vi "UHR-Fleezers Control (host) - 10.9.vi"() -> ()   [LabVIEW 2011] (continued)
                  n362 = local read "Oscillate Set 1"() -> (w595:bool)
                  n363 = local read "Stop All"() -> (w593:bool)
                  n364 = Or(x=w595, y=w590) -> (x .or. y?=w592:bool)
                  n365 = Not(x=w592) -> (.not. x?=w594:bool)
                  n366 = Compound Arithmetic op=OR(w593, w594) -> (w591:bool)
                }
              }
              n367 = node-c288() -> ()  [unwired: 2 out]
            }
            n368 = node-c288(w436) -> ()  [unwired: 1 out]
          }
        }
      }
      event "Fl. Triggered...": Value Change {
        n369 = event-data() -> ()  [unwired: 7 out]
        n370 = case shown="True" "Fl. Triggered..." {
          frame False {
          }
          frame True {
            n371 = node-c288() -> (w606:T21)  [unwired: 4 out]
            n372 = timed-loop {
              timing: w606 -> [_]
              timing-out: [_] -> w605
              tunnel: "Action" -> [w614]
              shift-right: [w611] -> _
              shift-left: u8 255 -> [w613]
              shift-right: [w608] -> _
              shift-left: 255 -> [w610]
              stop <- w607 stop-if-true
              n373 = node-c288() -> ()  [unwired: 2 out]
              n374 = flat-sequence {
                tunnel: w614 -> [w631]
                tunnel: w613 -> [w630]
                tunnel: [w629] -> w612
                tunnel: w610 -> [w616]
                tunnel: [w615] -> w609
                tunnel: [w911] -> w607
                tunnel: w612 -> [w910]
                tunnel: [w910] -> w611
                tunnel: [w909] -> w608
                tunnel: w609 -> [w909]
                frame #0 {
                  n375 = local read "Delta Fl. 2"() -> (w628:dbl)
                  n376 = local read "Delta Fl. 1"() -> (w623:dbl)
                  n377 = Multiply(x="Fl. Delta Thresh. (kHz)", y=1000.0) -> (x*y=w618:dbl)
                  n378 = Select(t=w623, s="APD to Watch", f=w628) -> (s? t:f=w619:dbl)
                  n379 = Greater?(x=w619, y=w618) -> (0:w624:bool)
                  n380 = Or(x="Force Yank", y=w624) -> (x .or. y?=w622:bool)
                  n381 = And(x=w622, y="Yank when bind or unbind?") -> (x .and. y?=w620:bool)
                  n382 = case shown="False" w620 {
                    tunnel: w631 -> [w633 w785]
                    tunnel: w630 -> [w635 w781]
                    tunnel: [w635 w778] -> w629
                    tunnel: w619 -> [w641 _]
                    tunnel: w618 -> [w640 _]
                    tunnel: "Force Yank" -> [w638 _]
                    tunnel: w616 -> [w637 w777]
                    tunnel: [w636 w777] -> w615
                    frame False {
                      n383 = Negate(x=w640) -> (-x=w632:dbl)
                      n384 = Less?(x=w641, y=w632) -> (x < y?=w639:bool)
                      n385 = Or(x=w638, y=w639) -> (x .or. y?=w634:bool)
                      n386 = case shown="True" w634 {
                        tunnel: w637 -> [w642 w652]
                        tunnel: [w642 w651] -> w636
                        tunnel: w633 -> [_ w650]
                        frame False {
                        }
                        frame True {
                          n387 = flat-sequence {
                            tunnel: w652 -> [w658]
                            tunnel: w650 -> [w655]
                            tunnel: [w657] -> w649
                            tunnel: [w656] -> w648
                            tunnel: [w655] -> w647
                            tunnel: w646 -> [w654]
                            tunnel: [w654] -> w645
                            tunnel: w644 -> [w653]
                            tunnel: [w653] -> w643
                            tunnel: [w704] -> w651
                            tunnel: w649 -> [w704]
                            tunnel: w648 -> [w703]
                            tunnel: w647 -> [w702]
                            tunnel: w645 -> [w701]
                            tunnel: w643 -> [w700]
                            frame #0 {
                              n388 = call <vilib>:"Beep.vi"() -> ()  [unwired: 12 in]
                              n389 = local write "Waiting"(FALSE ("Waiting")) -> ()
                              n390 = Increment(x=w658) -> (x+1=w657:i32)
                              n391 = case shown="\"Yank\"" w655 {
                                tunnel: w657 -> [_ w663 _]
                                frame "Alarm", Default {
                                }
                                frame "Yank" {
                                n392 = flat-sequence {
                                tunnel: w663 -> [w666]
                                tunnel: [w665] -> w662
                                tunnel: [w664] -> w661
                                tunnel: w662 -> [w676]
                                tunnel: w661 -> [w677]
                                frame #0 {
                                n393 = local read "Yank Delay (s)"() -> (w669:dbl)
                                n394 = local read "N Array El"() -> (w664:u8)
                                n395 = Quotient & Remainder(x=w666, y=w664) -> (x-y*floor(x/y)=w665:i32)  [unwired: 1 out]
                                n396 = Multiply(x=w669, y=1000.0) -> (x*y=w667:dbl)
                                n397 = Wait (ms)(milliseconds to wait=w667) -> ()  [unwired: 1 out]
                                }
                                frame #1 {
                                n398 = local read "Yank to which?"() -> (w671:bool)
                                n399 = local read "Random Choice"() -> (w681:bool)
                                n400 = local read "Yank to Delta Array (MHz)"() -> (w674:dbl[])
                                n401 = local read "Yank to SP"() -> (w675:dbl[])
                                n402 = Random Number (0-1)() -> (number: 0 to 1=w680:dbl)
                                n403 = Multiply(x=w677, y=w680) -> (x*y=w679:dbl)
                                n404 = Round Toward -Infinity(1:w679) -> (0:w678:dbl)
                                n405 = Select(t=w678, s=w681, f=w676) -> (s? t:f=w672:dbl)
                                n406 = Select(t=w674, s=w671, f=w675) -> (s? t:f=w673:dbl[])
                                n407 = Index Array(array=w673, index=w672) -> (element=w670:dbl)
                                n408 = case shown="False" w671 {
                                tunnel: w670 -> [w682 w697]
                                frame False {
                                n409 = flat-sequence {
                                tunnel: w682 -> [w683]
                                frame #0 {
                                n410 = property on="Trap Pos FB SP" class="DigNum (strict)"("Val(Sgnl)"=w683) -> ()  [unwired: 2 in, 2 out]
                                }
                                frame #1 {
                                n411 = Wait (ms)(milliseconds to wait=u32 700) -> ()  [unwired: 1 out]
                                }
                                frame #2 {
                                n412 = local read "Action (%)"() -> (w688:dbl)
                                n413 = Absolute Value(x=w688) -> (abs(x)=w687:dbl)
                                n414 = Greater?(x=w687, y=70.0) -> (0:w685:bool)
                                n415 = property on="Remove Action Offset" class="Bool (strict)"("Val(Sgnl)"=w685) -> ()  [unwired: 2 in, 2 out]
                                }
                                frame #3 {
                                n416 = for {
                                N: 4 -> [_]
                                n417 = flat-sequence {
                                frame #0 {
                                n418 = Wait (ms)(milliseconds to wait=u32 500) -> ()  [unwired: 1 out]
                                }
                                frame #1 {
                                n419 = local read "Action (%)"() -> (w694:dbl)
                                n420 = Absolute Value(x=w694) -> (abs(x)=w693:dbl)
                                n421 = Greater?(x=w693, y=70.0) -> (0:w691:bool)
                                n422 = property on="Remove Action Offset" class="Bool (strict)"("Val(Sgnl)"=w691) -> ()  [unwired: 2 in, 2 out]
                                }
                                }
                                }
                                }
                                frame #4 {
                                n423 = Wait (ms)(milliseconds to wait=u32 1500) -> ()  [unwired: 1 out]
                                }
                                frame #5 {
                                n424 = property on="Rem fb disp offset" class="Bool (strict)"("Val(Sgnl)"=TRUE ("Value (Signaling)")) -> ()  [unwired: 2 in, 2 out]
                                }
                                }
                                }
                                frame True {
                                n425 = property on="Trap Delta (MHz)" class="DigNum (strict)"("Val(Sgnl)"=w697) -> ()  [unwired: 2 in, 2 out]
                                }
                                }
                                }
                                }
                                }
                                frame "Image" {
                                n426 = property on="Confocal Image" class="Bool (strict)"("Val(Sgnl)"=TRUE ("Value (Signaling)")) -> ()  [unwired: 2 in, 2 out]
                                }
                              }
                              n427 = local write "Fl. High"(FALSE ("Fl. High")) -> ()
                              n428 = local read "Time (s)"() -> (w656:dbl)
                            }
                            frame #1 {
                              n429 = case shown="True" "Auto F Reset" {
                                tunnel: w703 -> [_ w708]
                                tunnel: w702 -> [_ w707]
                                tunnel: w701 -> [_ w706]
                                tunnel: w700 -> [_ w705]
                                frame False {
                                }
                                frame True {
                                n430 = node-c288() -> (w710:T21)  [unwired: 4 in]
                                n431 = timed-loop {
                                timing: w710 -> [_]
                                timing-out: [_] -> w709
                                tunnel: w708 -> [w715]
                                tunnel: w707 -> [w714]
                                tunnel: w706 -> [w713]
                                tunnel: w705 -> [w712]
                                stop <- w711 stop-if-true
                                n432 = node-c288() -> ()  [unwired: 1 in, 1 out]
                                n433 = local read "Fl. Delta Thresh. (kHz)"() -> (w724:dbl)
                                n434 = local read "APD to Watch"() -> (w725:bool)
                                n435 = local read "Delta Fl. 1"() -> (w726:dbl)
                                n436 = local read "Delta Fl. 2"() -> (w727:dbl)
                                n437 = local read "Fl. Triggered..."() -> (w718:bool)
                                n438 = local read "Stop All"() -> (w719:bool)
                                n439 = local read "Force Reset"() -> (w717:bool)
                                n440 = Multiply(x=w724, y=1000.0) -> (x*y=w722:dbl)
                                n441 = Not(x=w718) -> (.not. x?=w716:bool)
                                n442 = Select(t=w726, s=w725, f=w727) -> (s? t:f=w721:dbl)
                                n443 = Greater?(x=w721, y=w722) -> (0:w720:bool)
                                n444 = Compound Arithmetic op=OR(w720, w719, w716, w717) -> (w711:bool)
                                n445 = case shown="True" w711 {
                                tunnel: w715 -> [_ w731]
                                tunnel: w714 -> [_ w735]
                                tunnel: w713 -> [_ w734]
                                tunnel: w712 -> [_ w733]
                                frame False {
                                }
                                frame True {
                                n446 = case shown="\"Yank\"" w735 {
                                tunnel: w734 -> [_ w745]
                                tunnel: w733 -> [_ w743]
                                frame "Image", Default {
                                }
                                frame "Yank" {
                                n447 = flat-sequence {
                                tunnel: [w748] -> w746
                                tunnel: w745 -> [w748]
                                tunnel: [w747] -> w744
                                tunnel: w743 -> [w747]
                                tunnel: w746 -> [w754]
                                tunnel: w744 -> [w752]
                                frame #0 {
                                n448 = local read "Yank Delay (s)"() -> (w751:dbl)
                                n449 = Multiply(x=w751, y=1000.0) -> (x*y=w749:dbl)
                                n450 = Wait (ms)(milliseconds to wait=w749) -> ()  [unwired: 1 out]
                                }
                                frame #1 {
                                n451 = local read "Yank to which?"() -> (w753:bool)
                                n452 = case shown="False" w753 {
                                tunnel: w754 -> [_ w770]
                                tunnel: w752 -> [w755 _]
                                frame False {
                                n453 = flat-sequence {
                                tunnel: w755 -> [w756]
                                frame #0 {
                                n454 = property on="Trap Pos FB SP" class="DigNum (strict)"("Val(Sgnl)"=w756) -> ()  [unwired: 2 in, 2 out]
                                }
                                frame #1 {
                                n455 = Wait (ms)(milliseconds to wait=u32 700) -> ()  [unwired: 1 out]
                                }
                                frame #2 {
                                n456 = local read "Action (%)"() -> (w761:dbl)
                                n457 = Absolute Value(x=w761) -> (abs(x)=w760:dbl)
                                n458 = Greater?(x=w760, y=70.0) -> (0:w758:bool)
                                n459 = property on="Remove Action Offset" class="Bool (strict)"("Val(Sgnl)"=w758) -> ()  [unwired: 2 in, 2 out]
                                }
                                frame #3 {
                                n460 = for {
                                N: 4 -> [_]
                                n461 = flat-sequence {
                                frame #0 {
                                n462 = Wait (ms)(milliseconds to wait=u32 500) -> ()  [unwired: 1 out]
                                }
                                frame #1 {
                                n463 = local read "Action (%)"() -> (w767:dbl)
                                n464 = Absolute Value(x=w767) -> (abs(x)=w766:dbl)
                                n465 = Greater?(x=w766, y=70.0) -> (0:w764:bool)
                                n466 = property on="Remove Action Offset" class="Bool (strict)"("Val(Sgnl)"=w764) -> ()  [unwired: 2 in, 2 out]
                                }
                                }
                                }
                                }
                                frame #4 {
                                n467 = Wait (ms)(milliseconds to wait=u32 1500) -> ()  [unwired: 1 out]
                                }
                                frame #5 {
                                n468 = property on="Rem fb disp offset" class="Bool (strict)"("Val(Sgnl)"=TRUE ("Value (Signaling)")) -> ()  [unwired: 2 in, 2 out]
                                }
                                }
                                }
                                frame True {
                                n469 = property on="Trap Delta (MHz)" class="DigNum (strict)"("Val(Sgnl)"=w770) -> ()  [unwired: 2 in, 2 out]
                                }
                                }
                                }
                                }
                                }
                                }
                                n470 = local read "Time (s)"() -> (w730:dbl)
                                n471 = Subtract(x=w731, y=w730) -> (x-y=w742:dbl)
                                n472 = Number To Decimal String(number=w742, width (-)=i16 0) -> (decimal integer string=w740:string)
                                n473 = Concatenate Strings(w740, " s fluorescence event") -> (w737:string)
                                n474 = local read "Messages"() -> (w738:string)
                                n475 = local write "Duration (s)"(w742) -> ()
                                n476 = call "Update messages.vi"("Message to add"=w737, "Old message string"=w738) -> ("New message string"=w736:string)
                                n477 = local write "Messages"(w736) -> ()
                                n478 = call <vilib>:"Beep.vi"() -> ()  [unwired: 12 in]
                                n479 = local write "Force Reset"(FALSE ("Force Reset")) -> ()
                                n480 = local write "Fl. High"(TRUE ("Fl. High")) -> ()
                                n481 = local write "Waiting"(TRUE ("Waiting")) -> ()
                                }
                                }
                                n482 = node-c288() -> ()  [unwired: 1 in, 1 out]
                                }
                                n483 = node-c288(w709) -> ()  [unwired: 1 out]
                                }
                              }
                            }
                          }
                          n484 = local read "Trap Delta (MHz)"() -> (w646:dbl)
                          n485 = local read "Trap Pos FB SP"() -> (w644:fxp<+/-,16,1>)
                        }
                      }
                    }
                    frame True {
                      n486 = flat-sequence {
                        tunnel: w782 -> [w792]
                        tunnel: [w792] -> w786
                        tunnel: w785 -> [w791]
                        tunnel: [w791] -> w784
                        tunnel: [w790] -> w783
                        tunnel: w781 -> [w789]
                        tunnel: [w788] -> w780
                        tunnel: w776 -> [w787]
                        tunnel: [w787] -> w775
                        tunnel: w786 -> [w838]
                        tunnel: w784 -> [w837]
                        tunnel: w783 -> [w836]
                        tunnel: w780 -> [w835]
                        tunnel: [w835] -> w779
                        tunnel: w775 -> [w834]
                        tunnel: w779 -> [w907]
                        tunnel: [w907] -> w778
                        frame #0 {
                          n487 = call <vilib>:"Beep.vi"() -> ()  [unwired: 3 in, 9 out]
                          n488 = local write "Waiting"(FALSE ("Waiting")) -> ()
                          n489 = Increment(x=w789) -> (x+1=w788:u8)
                          n490 = case shown="\"Yank\"" w791 {
                            tunnel: w788 -> [_ _ w798]
                            frame "Image" {
                              n491 = property on="Confocal Image" class="Bool (strict)"("Val(Sgnl)"=TRUE ("Value (Signaling)")) -> ()  [unwired: 2 in, 2 out]
                            }
                            frame "Alarm", Default {
                            }
                            frame "Yank" {
                              n492 = flat-sequence {
                                tunnel: w798 -> [w801]
                                tunnel: [w800] -> w797
                                tunnel: ["N Array El"] -> w796
                                tunnel: w797 -> [w815]
                                tunnel: w796 -> [w811]
                                frame #0 {
                                n493 = Multiply(x="Yank Delay (s)", y=1000.0) -> (x*y=w804:dbl)
                                n494 = Quotient & Remainder(x=w801, y="N Array El") -> (x-y*floor(x/y)=w800:u8)  [unwired: 1 out]
                                n495 = Wait (ms)(milliseconds to wait=w804) -> ()  [unwired: 1 out]
                                }
                                frame #1 {
                                n496 = Random Number (0-1)() -> (number: 0 to 1=w812:dbl)
                                n497 = Multiply(x=w811, y=w812) -> (x*y=w810:dbl)
                                n498 = Round Toward -Infinity(1:w810) -> (0:w809:dbl)
                                n499 = Select(t=w809, s="Random Choice", f=w815) -> (s? t:f=w813:dbl)
                                n500 = Select(t="Yank to Delta Array (MHz)", s="Yank to which?", f="Yank to SP") -> (s? t:f=w806:dbl[])
                                n501 = Index Array(array=w806, index=w813) -> (element=w816:dbl)
                                n502 = case shown="False" "Yank to which?" {
                                tunnel: w816 -> [w817 w832]
                                frame False {
                                n503 = flat-sequence {
                                tunnel: w817 -> [w818]
                                frame #0 {
                                n504 = property on="Trap Pos FB SP" class="DigNum (strict)"("Val(Sgnl)"=w818) -> ()  [unwired: 2 in, 2 out]
                                }
                                frame #1 {
                                n505 = Wait (ms)(milliseconds to wait=u32 700) -> ()  [unwired: 1 out]
                                }
                                frame #2 {
                                n506 = local read "Action (%)"() -> (w823:dbl)
                                n507 = Absolute Value(x=w823) -> (abs(x)=w822:dbl)
                                n508 = Greater?(x=w822, y=70.0) -> (0:w820:bool)
                                n509 = property on="Remove Action Offset" class="Bool (strict)"("Val(Sgnl)"=w820) -> ()  [unwired: 2 in, 2 out]
                                }
                                frame #3 {
                                n510 = for {
                                N: 4 -> [_]
                                n511 = flat-sequence {
                                frame #0 {
                                n512 = Wait (ms)(milliseconds to wait=u32 500) -> ()  [unwired: 1 out]
                                }
                                frame #1 {
                                n513 = local read "Action (%)"() -> (w829:dbl)
                                n514 = Absolute Value(x=w829) -> (abs(x)=w828:dbl)
                                n515 = Greater?(x=w828, y=70.0) -> (0:w826:bool)
                                n516 = property on="Remove Action Offset" class="Bool (strict)"("Val(Sgnl)"=w826) -> ()  [unwired: 2 in, 2 out]
                                }
                                }
                                }
                                }
                                frame #4 {
                                n517 = Wait (ms)(milliseconds to wait=u32 1500) -> ()  [unwired: 1 out]
                                }
                                frame #5 {
                                n518 = property on="Rem fb disp offset" class="Bool (strict)"("Val(Sgnl)"=TRUE ("Value (Signaling)")) -> ()  [unwired: 2 in, 2 out]
                                }
                                }
                                }
                                frame True {
                                n519 = property on="Trap Delta (MHz)" class="DigNum (strict)"("Val(Sgnl)"=w832) -> ()  [unwired: 2 in, 2 out]
                                }
                                }
                                }
                              }
                            }
                          }
                          n520 = local read "Time (s)"() -> (w790:dbl)
                          "Fl. High" <- TRUE ("Yanking")
                        }
                        frame #1 {
                          n521 = local read "Auto F Reset"() -> (w833:bool)
                          n522 = case shown="True" w833 {
                            tunnel: w838 -> [_ w842]
                            tunnel: w837 -> [_ w841]
                            tunnel: w836 -> [_ w840]
                            tunnel: w834 -> [_ w839]
                            frame False {
                            }
                            frame True {
                              n523 = node-c288() -> (w844:T21)  [unwired: 4 out]
                              n524 = timed-loop {
                                timing: w844 -> [_]
                                timing-out: [_] -> w843
                                tunnel: w842 -> [w862]
                                tunnel: w841 -> [w861]
                                tunnel: w840 -> [w860]
                                tunnel: w839 -> [w859]
                                stop <- w845 stop-if-true
                                n525 = node-c288() -> ()  [unwired: 2 out]
                                n526 = local read "Fl. Delta Thresh. (kHz)"() -> (w853:dbl)
                                n527 = local read "Fl. Triggered..."() -> (w858:bool)
                                n528 = local read "Delta Fl. 1"() -> (w849:dbl)
                                n529 = local read "Delta Fl. 2"() -> (w847:dbl)
                                n530 = local read "Stop All"() -> (w856:bool)
                                n531 = local read "APD to Watch"() -> (w848:bool)
                                n532 = Select(t=w849, s=w848, f=w847) -> (s? t:f=w846:dbl)
                                n533 = Not(x=w858) -> (.not. x?=w857:bool)
                                n534 = Multiply(x=w853, y=1000.0) -> (x*y=w852:dbl)
                                n535 = Negate(x=w852) -> (-x=w851:dbl)
                                n536 = Less?(x=w846, y=w851) -> (x < y?=w855:bool)
                                n537 = Compound Arithmetic op=OR(w855, w856, w857, "Force Reset") -> (w845:bool)
                                n538 = case shown="True" w845 {
                                tunnel: w862 -> [_ w874]
                                tunnel: w861 -> [_ w873]
                                tunnel: w860 -> [_ w863]
                                tunnel: w859 -> [_ w865]
                                frame False {
                                }
                                frame True {
                                n539 = case shown="\"Yank\"" w873 {
                                tunnel: w874 -> [_ w877]
                                tunnel: w865 -> [_ w875]
                                frame "Image", Default {
                                }
                                frame "Yank" {
                                n540 = flat-sequence {
                                tunnel: [w883] -> w878
                                tunnel: w877 -> [w883]
                                tunnel: [w879] -> w876
                                tunnel: w875 -> [w879]
                                tunnel: w878 -> [w886]
                                tunnel: w876 -> [w884]
                                frame #0 {
                                n541 = local read "Yank Delay (s)"() -> (w882:dbl)
                                n542 = Multiply(x=w882, y=1000.0) -> (x*y=w880:dbl)
                                n543 = Wait (ms)(milliseconds to wait=w880) -> ()  [unwired: 1 out]
                                }
                                frame #1 {
                                n544 = local read "Yank to which?"() -> (w885:bool)
                                n545 = case shown="False" w885 {
                                tunnel: w886 -> [_ w902]
                                tunnel: w884 -> [w887 _]
                                frame False {
                                n546 = flat-sequence {
                                tunnel: w887 -> [w888]
                                frame #0 {
                                n547 = property on="Trap Pos FB SP" class="DigNum (strict)"("Val(Sgnl)"=w888) -> ()  [unwired: 2 in, 2 out]
                                }
                                frame #1 {
                                n548 = Wait (ms)(milliseconds to wait=u32 700) -> ()  [unwired: 1 out]
                                }
                                frame #2 {
                                n549 = local read "Action (%)"() -> (w893:dbl)
                                n550 = Absolute Value(x=w893) -> (abs(x)=w892:dbl)
                                n551 = Greater?(x=w892, y=70.0) -> (0:w890:bool)
                                n552 = property on="Remove Action Offset" class="Bool (strict)"("Val(Sgnl)"=w890) -> ()  [unwired: 2 in, 2 out]
                                }
                                frame #3 {
                                n553 = for {
                                N: 4 -> [_]
                                n554 = flat-sequence {
                                frame #0 {
                                n555 = Wait (ms)(milliseconds to wait=u32 500) -> ()  [unwired: 1 out]
                                }
                                frame #1 {
                                n556 = local read "Action (%)"() -> (w899:dbl)
                                n557 = Absolute Value(x=w899) -> (abs(x)=w898:dbl)
                                n558 = Greater?(x=w898, y=70.0) -> (0:w896:bool)
                                n559 = property on="Remove Action Offset" class="Bool (strict)"("Val(Sgnl)"=w896) -> ()  [unwired: 2 in, 2 out]
                                }
                                }
                                }
                                }
                                frame #4 {
                                n560 = Wait (ms)(milliseconds to wait=u32 1500) -> ()  [unwired: 1 out]
                                }
                                frame #5 {
                                n561 = property on="Rem fb disp offset" class="Bool (strict)"("Val(Sgnl)"=TRUE ("Value (Signaling)")) -> ()  [unwired: 2 in, 2 out]
                                }
                                }
                                }
                                frame True {
                                n562 = property on="Trap Delta (MHz)" class="DigNum (strict)"("Val(Sgnl)"=w902) -> ()  [unwired: 2 in, 2 out]
                                }
                                }
                                }
                                }
                                }
                                }
                                n563 = local read "Time (s)"() -> (w864:dbl)
                                n564 = local read "Messages"() -> (w872:string)
                                n565 = Subtract(x=w864, y=w863) -> (x-y=w870:dbl)
                                "Duration (s)" <- w870
                                n566 = Number To Decimal String(number=w870, width (-)=i16 0) -> (decimal integer string=w868:string)
                                n567 = Concatenate Strings(w868, " s fluorescence event." ("string")) -> (w866:string)
                                n568 = call "Update messages.vi"("Message to add"=w866, "Old message string"=w872) -> ("New message string"=w871:string)
                                n569 = local write "Messages"(w871) -> ()
                                n570 = call <vilib>:"Beep.vi"() -> ()  [unwired: 3 in, 9 out]
                                }
                                }
                                n571 = node-c288() -> ()  [unwired: 2 out]
                              }
                              n572 = node-c288(w843) -> ()  [unwired: 1 out]
                            }
                          }
                        }
                        frame #2 {
                          n573 = local write "Fl. High"(FALSE ("Yanking")) -> ()
                        }
                      }
                      n574 = local read "Trap Delta (MHz)"() -> (w782:dbl)
                      n575 = local read "Trap Pos FB SP"() -> (w776:fxp<+/-,16,1>)
                    }
                  }
                }
                frame #1 {
                  n576 = local read "Stop All"() -> (w914:bool)
                  n577 = local read "Fl. Triggered..."() -> (w912:bool)
                  n578 = Not(x=w912) -> (.not. x?=w913:bool)
                  n579 = Or(x=w913, y=w914) -> (x .or. y?=w911:bool)
                  n580 = Not(x=w911) -> (.not. x?=→"Waiting":bool)
                }
              }
              n581 = node-c288() -> ()  [unwired: 2 out]
            }
            n582 = node-c288(w605) -> ()  [unwired: 1 out]
          }
        }
      }
      event "Stop All": Value Change {
        n583 = event-data() -> ()  [unwired: 7 out]
        n584 = local read "Stop All"() -> (w920:bool)
      }
    }
    n585 = node-c288() -> ()  [unwired: 2 out]
  }
  n586 = node-c288() -> (w79:T21)  [unwired: 4 in]
  n587 = node-c288(2 ("Processor")) -> (w92:T21)  [unwired: 3 out]
  n588 = timed-loop "Run Scripts, including: stage motion" {
    tunnel: w84 -> [w927]
    tunnel: w83 -> [w928]
    tunnel: [w928] -> w82
    tunnel: [w927] -> w81
    timing: w79 -> [_]
    timing-out: [_] -> w78
    tunnel: w64 -> [w926]
    tunnel: w65 -> [w925]
    tunnel: w4 -> [w922]
    tunnel: w3 -> [w921]
    tunnel: w2 -> [w923]
    tunnel: w1 -> [w924]
    stop <- w929 stop-if-true
    n589 = node-c288() -> ()  [unwired: 1 in, 1 out]
    n590 = event shown="[12] \"Force FB Data\nScript\": Value Change" {
      selector: _ -> [_ _ _ _ _ _ _ _ _ _ _ _ _ _ _ _ _ _ _]
      dyn-events: _ -> [_ _ _ _ _ _ _ _ _ _ _ _ _ _ _ _ _ _ _]
      timeout: _ -> [_ _ _ _ _ _ _ _ _ _ _ _ _ _ _ _ _ _ _]
      tunnel: ["Set Position" "Move to Position" _ _ "Read Harvard" _ _ _ _ _ _ "Got ADig bead" "Force FB Data\nScript" _ "Got DNA bead" "Take Stepping Data" _ "Take Detection Laser\nImage" _] -> _
      tunnel: [_ _ _ _ _ _ _ _ _ _ _ _ _ _ _ _ _ _ w1546] -> w929
      tunnel: w927 -> [w947 w955 w968 w998 _ w1043 w1083 w1164 w1193 w1325 w1351 _ w1387 _ _ _ _ _ _]
      tunnel: w928 -> [w948 w956 w969 w999 _ w1044 w1084 w1165 w1194 w1326 w1352 _ w1388 _ _ _ _ _ _]
      tunnel: w926 -> [_ _ _ _ w1028 _ _ _ _ _ _ _ _ _ _ _ _ _ _]
      tunnel: w925 -> [_ _ _ _ w1027 _ _ _ _ _ _ _ _ _ _ _ _ _ _]
      tunnel: w924 -> [_ _ _ _ _ _ _ _ _ _ _ _ _ _ _ _ _ _ _]
      tunnel: w923 -> [_ _ _ _ _ _ _ _ _ _ _ _ _ _ _ _ _ _ _]
      tunnel: w922 -> [_ _ _ _ _ _ _ _ _ _ _ _ _ _ _ _ _ _ _]
      tunnel: w921 -> [_ _ _ _ _ _ _ _ _ _ _ _ _ _ _ _ _ _ _]
      event "Set Position", "Set Position 2", "Set Position 3", "Set Position 4", "Set Position 5", "Set Position 1": Value Change {
        n591 = event-data() -> ()  [unwired: 1 in, 5 out]
        n592 = Build Array("Set Position 1", "Set Position 2", "Set Position 3", "Set Position 4", "Set Position 5") -> (w946:bool[])
        n593 = Boolean Array To Number(Boolean array=w946) -> (number=w945:u32)
        n594 = Logarithm Base 2(1:w945) -> (0:w937:dbl)
        n595 = call "Read Stage Position.vi"("error in"=w947, "VISA resource name in"=w948) -> ("Current Position"=w952:cluster{dbl, dbl, dbl}, "error out"=w951:errorcluster)  [unwired: 2 out]
        n596 = Decrement(x="Position") -> (x-1=w935:dbl)
        n597 = Greater Or Equal?(x=w937, y=0.0) -> (x >= y?=w938:bool)
        n598 = Cluster To Array(cluster=w952) -> (array=w949:dbl[])
        n599 = local write "Stage Control Serial Error"(w951) -> ()
        n600 = Select(t=w937, s=w938, f=w935) -> (s? t:f=w934:dbl)
        n601 = Increment(x=w934) -> (x+1=w933:dbl)
        n602 = Build Array (concatenate)(w933, w949) -> (w932:dbl[])
        n603 = Replace Array Subset(array="Saved Stage Positions", new element=w932, index (row)=w934) -> (w950:dbl[][])  [unwired: 1 in]
        n604 = local write "Saved Stage Positions"(w950) -> ()
      }
      event "Move to Position": Value Change {
        n605 = event-data() -> ()  [unwired: 1 in, 5 out]
        n606 = flat-sequence {
          tunnel: w956 -> [w960]
          tunnel: w955 -> [w959]
          frame #0 {
            n607 = local read "Saved Stage Positions"() -> (w962:dbl[][])
            n608 = local read "Position"() -> (w961:dbl)
            n609 = local write "Stage Moving"(TRUE ("Stage Moving")) -> ()
            n610 = call "move to saved stage position.vi"("error in"=w959, "Stage VISA resource name in"=w960, "Position"=w961, "Saved Stage Positions"=w962) -> ("error out"=w958:errorcluster)  [unwired: 1 out]
            n611 = local write "Stage Control Serial Error"(w958) -> ()
          }
          frame #1 {
            n612 = call <vilib>:"Beep.vi"() -> ()  [unwired: 3 in, 9 out]
            n613 = local write "Stage Moving"(FALSE ("Stage Moving")) -> ()
          }
        }
      }
      event "Move Cap. 1 (DNA Bottom)": Value Change {
        n614 = event-data() -> ()  [unwired: 1 in, 5 out]
        n615 = local write "Move Cap. 1 (DNA Bottom)"(FALSE ("Move Cap. 1 (DNA Right)")) -> ()
        n616 = flat-sequence {
          tunnel: w968 -> [w971]
          tunnel: w969 -> [w972]
          tunnel: [w972] -> w966
          tunnel: [w971] -> w965
          tunnel: w966 -> [w974]
          tunnel: w965 -> [w973]
          frame #0 {
            n617 = property on="Sample Channel\nFlow" class="Bool (strict)"("Val(Sgnl)"="Cap 1 Samp Flow ON") -> ()  [unwired: 2 in, 2 out]
          }
          frame #1 {
            n618 = local read "Saved Stage Positions"() -> (w984:dbl[][])
            n619 = local write "Stage Moving"(TRUE ("Stage Moving")) -> ()
            n620 = Array Subset(array=w984, index (row)=0 ("index"), length (row)=1 ("length"), index (col)=1 ("index"), length (col)=3 ("length")) -> (w981:dbl[][])
            n621 = Reshape Array(w981, 3 ("dimension size")) -> (w979:dbl[])
            n622 = Array To Cluster(array=w979) -> (cluster=w978:cluster{"[0]":dbl, "[1]":dbl, "[2]":dbl})
            n623 = call "Set Stage Position.vi"("Position"=w978, "error in"=w973, "VISA resource name in"=w974) -> ("error out"=w977:errorcluster)  [unwired: 2 out]
            n624 = local write "Stage Control Serial Error"(w977) -> ()
          }
          frame #2 {
            n625 = local write "Stage Moving"(FALSE ("Stage Moving")) -> ()
            n626 = case shown="True" "Cap 1 Flow ON" {
              frame False {
              }
              frame True {
                n627 = property on="Inject Pump 1" class="Bool (strict)"("Val(Sgnl)"=TRUE ("Value (Signaling)")) -> ()  [unwired: 2 in, 2 out]
              }
            }
            n628 = call <vilib>:"Beep.vi"() -> ()  [unwired: 3 in, 9 out]
          }
          frame #3 {
            n629 = property on="Sample Channel\nFlow" class="Bool (strict)"("Val(Sgnl)"=FALSE ("Value (Signaling)")) -> ()  [unwired: 2 in, 2 out]
            n630 = local read "Cap. 2 BD T1?\n(ADig T1, DNA T2)"() -> (w991:bool)
            n631 = case shown="True" w991 {
              tunnel: "Cap 1 T ON" -> [w993 w994]
              frame False {
                n632 = property on="Trap 1 (ON/OFF)" class="Bool (strict)"("Val(Sgnl)"=w993) -> ()  [unwired: 2 in, 2 out]
              }
              frame True {
                n633 = property on="Trap 2 (ON/OFF)" class="Bool (strict)"("Val(Sgnl)"=w994) -> ()  [unwired: 2 in, 2 out]
              }
            }
            n634 = property on="Got DNA bead" class="Bool"("Key Focus"=TRUE) -> ()  [unwired: 2 in, 2 out]
          }
        }
      }
      event "Move Cap. 2 (ADig Top)": Value Change {
        n635 = event-data() -> ()  [unwired: 1 in, 5 out]
        n636 = local write "Move Cap. 2 (ADig Top)"(FALSE ("Move Cap. 2 (ADig Left)")) -> ()
        n637 = flat-sequence {
          tunnel: w998 -> [w1001]
          tunnel: w999 -> [w1002]
          tunnel: [w1002] -> w996
          tunnel: [w1001] -> w995
          tunnel: w996 -> [w1005]
          tunnel: w995 -> [w1004]
          frame #0 {
            n638 = property on="Sample Channel\nFlow" class="Bool (strict)"("Val(Sgnl)"="Cap 2 Samp Flow ON") -> ()  [unwired: 2 in, 2 out]
          }
          frame #1 {
            w1003 = FALSE ("Value (Signaling)")
            n639 = local read "Saved Stage Positions"() -> (w1015:dbl[][])
            n640 = local write "Stage Moving"(TRUE ("Stage Moving")) -> ()
            n641 = Array Subset(array=w1015, index (row)=1 ("index"), length (row)=1 ("length"), index (col)=1 ("index"), length (col)=3 ("length")) -> (w1012:dbl[][])
            n642 = Reshape Array(w1012, 3 ("dimension size")) -> (w1010:dbl[])
            n643 = property on="Trap 1 (ON/OFF)" class="Bool (strict)"("Val(Sgnl)"=w1003) -> ()  [unwired: 2 in, 2 out]
            n644 = property on="Trap 1 (ON/OFF)" class="Bool (strict)"("Val(Sgnl)"=w1003) -> ()  [unwired: 2 in, 2 out]
            n645 = Array To Cluster(array=w1010) -> (cluster=w1009:cluster{"[0]":dbl, "[1]":dbl, "[2]":dbl})
            n646 = call "Set Stage Position.vi"("Position"=w1009, "error in"=w1004, "VISA resource name in"=w1005) -> ("error out"=w1008:errorcluster)  [unwired: 2 out]
            n647 = local write "Stage Control Serial Error"(w1008) -> ()
          }
          frame #2 {
            n648 = local write "Stage Moving"(FALSE ("Stage Moving")) -> ()
            n649 = call <vilib>:"Beep.vi"() -> ()  [unwired: 3 in, 9 out]
            n650 = case shown="True" "Cap 2 Flow ON" {
              frame False {
              }
              frame True {
                n651 = property on="Inject Pump 3" class="Bool (strict)"("Val(Sgnl)"=TRUE ("Value (Signaling)")) -> ()  [unwired: 2 in, 2 out]
              }
            }
          }
          frame #3 {
            n652 = property on="Sample Channel\nFlow" class="Bool (strict)"("Val(Sgnl)"=FALSE ("Value (Signaling)")) -> ()  [unwired: 2 in, 2 out]
            n653 = case shown="False" "Cap. 2 BD T1?\n(ADig T1, DNA T2)" {
              tunnel: "Cap 2 T ON" -> [w1024 w1025]
              frame False {
                n654 = property on="Trap 2 (ON/OFF)" class="Bool (strict)"("Val(Sgnl)"=w1024) -> ()  [unwired: 2 in, 2 out]
              }
              frame True {
                n655 = property on="Trap 1 (ON/OFF)" class="Bool (strict)"("Val(Sgnl)"=w1025) -> ()  [unwired: 2 in, 2 out]
              }
            }
            n656 = property on="Got ADig bead" class="Bool"("Key Focus"=TRUE) -> ()  [unwired: 2 in, 2 out]
          }
        }
      }
      event "Read Harvard": Value Change {
        n657 = event-data() -> ()  [unwired: 1 in, 5 out]
        n658 = Concatenate Strings("write buffer", "\r") -> (w1030:string)
        n659 = VISA Write(VISA resource name=w1028, write buffer=w1030, error in (no error)=w1027) -> (VISA resource name out=w1039:refnum<visa-resource-name>, error out=w1038:errorcluster)  [unwired: 1 out]
        n660 = stacked-sequence {
          tunnel: [w1042] -> w1037
          tunnel: w1039 -> [w1042]
          tunnel: w1038 -> [w1041]
          tunnel: [w1041] -> w1032
          frame #0 {
            n661 = Wait (ms)(milliseconds to wait=50) -> ()  [unwired: 1 out]
          }
        }
        n662 = property class="Instr"(reference=w1037, error in=w1032) -> (reference out=w1036:refnum<visa-resource-name>, error out=w1034:errorcluster, "Serial Settings:Number of Bytes at Serial Port"=w1035:u32)
        "Serial Settings:Number of Bytes at Serial Port" <- w1035
        n663 = VISA Read(VISA resource name=w1036, byte count=w1035, error in (no error)=w1034) -> (read buffer=w1033:string)  [unwired: 3 out]
        "read buffer" <- w1033
        n664 = Fract/Exp String To Number(string=w1033) -> ()  [unwired: 5 out]
      }
      event "+z", "-z": Value Change {
        n665 = event-data() -> ()  [unwired: 1 in, 5 out]
        n666 = flat-sequence {
          tunnel: w1043 -> [w1065]
          tunnel: w1044 -> [w1045]
          frame #0 {
            n667 = call "Read Stage Position.vi"("error in"=w1065, "VISA resource name in"=w1045) -> ("Current Position"=w1050:cluster{dbl, dbl, dbl}, "error out"=w1063:errorcluster, "VISA resource name out"=w1064:refnum<visa-resource-name>)  [unwired: 1 out]
            n668 = local read "Saved Stage Positions"() -> (w1074:dbl[][])
            n669 = Divide(x="z nudge increment (um)", y=1000.0) -> (x/y=w1062:dbl)
            n670 = Boolean To (0,1)(Boolean="+z") -> (0, 1=w1054:i16)
            n671 = Boolean To (0,1)(Boolean="-z") -> (0, 1=w1055:i16)
            n672 = Array Subset(array=w1074, index (row)=1 ("index"), length (row)=1 ("length"), index (col)=1 ("index"), length (col)=3 ("length")) -> (w1071:dbl[][])
            n673 = Multiply(x=w1054, y=w1062) -> (x*y=w1058:dbl)
            n674 = Multiply(x=w1055, y=w1062) -> (x*y=w1056:dbl)
            n675 = Unbundle(w1050) -> (w1048:dbl, w1047:dbl, w1051:dbl)
            n676 = Negate(x=w1056) -> (-x=w1057:dbl)
            n677 = Reshape Array(w1071, 3 ("dimension size")) -> (w1069:dbl[])
            n678 = Add(x=w1058, y=w1057) -> (x+y=w1059:dbl)
            n679 = Array To Cluster(array=w1069) -> ()  [unwired: 1 out]
            n680 = Add(x=w1059, y=w1051) -> (x+y=w1049:dbl)
            n681 = Bundle(cluster=w1050, w1048, w1047, w1049) -> (w1046:cluster{dbl, dbl, dbl})
            n682 = call "Set Stage Position.vi"("Position"=w1046, "error in"=w1063, "VISA resource name in"=w1064) -> ("error out"=w1068:errorcluster)  [unwired: 2 out]
            n683 = local write "Stage Moving"(TRUE ("Stage Moving")) -> ()
            n684 = local write "Stage Control Serial Error"(w1068) -> ()
          }
          frame #1 {
            n685 = local write "Stage Moving"(FALSE ("Stage Moving")) -> ()
            n686 = call <vilib>:"Beep.vi"() -> ()  [unwired: 3 in, 9 out]
          }
        }
      }
      event "Cal/Data Acq. Spot": Value Change {
        n687 = event-data() -> ()  [unwired: 1 in, 5 out]
        n688 = flat-sequence {
          tunnel: w1083 -> [w1087]
          tunnel: w1084 -> [w1088]
          tunnel: [w1088] -> w1080
          tunnel: [w1087] -> w1079
          tunnel: w1080 -> [w1093]
          tunnel: w1079 -> [w1092]
          tunnel: ["Cal @ (MHz)"] -> w1077
          tunnel: [w1097] -> w1081
          tunnel: w1077 -> [w1097]
          tunnel: w1081 -> [w1106]
          tunnel: ["W/ Offset 1"] -> w1078
          tunnel: w1081 -> [w1127]
          tunnel: w1078 -> [w1125]
          frame #0 {
            n689 = property on="Sample Channel\nFlow" class="Bool (strict)"("Val(Sgnl)"="Daq spot flow on") -> ()  [unwired: 2 in, 2 out]
            n690 = Wait (ms)(milliseconds to wait=u32 250) -> ()  [unwired: 1 out]
          }
          frame #1 {
            n691 = local read "Saved Stage Positions"() -> (w1090:dbl[][])
            n692 = property on="Trap Delta (MHz)" class="DigNum (strict)"("Val(Sgnl)"="Cal @ (MHz)") -> ()  [unwired: 2 in, 2 out]
            n693 = local write "Stage Moving"(TRUE ("Stage Moving")) -> ()
            n694 = call "move to saved stage position.vi"("error in"=w1092, "Stage VISA resource name in"=w1093, "Position"="Cal Stage Position", "Saved Stage Positions"=w1090) -> ("error out"=w1091:errorcluster)  [unwired: 1 out]
            n695 = local write "Stage Control Serial Error"(w1091) -> ()
          }
          frame #2 {
            n696 = local write "Stage Moving"(FALSE ("Stage Moving")) -> ()
            n697 = property on="Sample Channel\nFlow" class="Bool (strict)"("Val(Sgnl)"="Flow ON during cal?") -> ()  [unwired: 2 in, 2 out]
            n698 = call <vilib>:"Beep.vi"() -> ()  [unwired: 3 in, 9 out]
          }
          frame #3 {
            n699 = Wait (ms)(milliseconds to wait=u32 1000) -> ()  [unwired: 1 out]
          }
          frame #4 {
            n700 = property on="Save Calibration" class="Bool (strict)"("Val(Sgnl)"=TRUE ("Value (Signaling)")) -> ()  [unwired: 2 in, 2 out]
          }
          frame #5 {
            n701 = Wait (ms)(milliseconds to wait=u32 2000) -> ()  [unwired: 1 out]
          }
          frame #6 {
            # "Check to see if \nsaving done"
            n702 = while {
              stop <- w1102 stop-if-true
              n703 = local read "Saving..."() -> (w1103:bool)
              n704 = Wait (ms)(milliseconds to wait=u32 100) -> ()  [unwired: 1 out]
              n705 = Not(x=w1103) -> (.not. x?=w1102:bool)
            }
          }
          frame #7 {
            n706 = case shown="True" "W/ Offset 1" {
              tunnel: w1106 -> [_ w1107]
              frame False {
              }
              frame True {
                n707 = stacked-sequence {
                  tunnel: w1107 -> [_ _ _ _ _ _ _ w1124]
                  frame #0 {
                    n708 = property on="Trap Delta (MHz)" class="DigNum (strict)"("Val(Sgnl)"="Offset 1 Start (MHz)") -> ()  [unwired: 2 in, 2 out]
                    n709 = Replace Array Subset(array=u32[] [0] ("Index Values"), new element="Offset 1 Set", index=0) -> (w1108:u32[])
                    n710 = property on="Saved AOD Raster Scan Parameter Sets" class="Arr (strict)"("Index Values"=w1108) -> ()  [unwired: 2 in, 2 out]
                  }
                  frame #1 {
                    n711 = Wait (ms)(milliseconds to wait=u32 200) -> ()  [unwired: 1 out]
                  }
                  frame #2 {
                    n712 = property on="Load parameters" class="Bool (strict)"("Val(Sgnl)"=TRUE ("Value (Signaling)")) -> ()  [unwired: 2 in, 2 out]
                  }
                  frame #3 {
                    n713 = Wait (ms)(milliseconds to wait=u32 200) -> ()  [unwired: 1 out]
                  }
                  frame #4 {
                    n714 = property on="Trap Raster Scan" class="Bool (strict)"("Val(Sgnl)"=TRUE ("Value (Signaling)")) -> ()  [unwired: 2 in, 2 out]
                  }
                  frame #5 {
                    n715 = Wait (ms)(milliseconds to wait=u32 2000) -> ()  [unwired: 1 out]
                  }
                  frame #6 {
                    n716 = while {
                      stop <- w1121 stop-if-true
                      n717 = local read "Raster Scanning..."() -> (w1123:bool)
                      n718 = local read "Saving..."() -> (w1119:bool)
                      n719 = Wait (ms)(milliseconds to wait=u32 100) -> ()  [unwired: 1 out]
                      n720 = Not(x=w1119) -> (.not. x?=w1118:bool)
                      n721 = Not(x=w1123) -> (.not. x?=w1120:bool)
                      n722 = And(x=w1120, y=w1118) -> (x .and. y?=w1121:bool)
                    }
                  }
                  frame #7 {
                    n723 = property on="Trap Delta (MHz)" class="DigNum (strict)"("Val(Sgnl)"=w1124) -> ()  [unwired: 2 in, 2 out]
                  }
                }
              }
            }
          }
          frame #8 {
            n724 = local read "Save ave N"() -> (w1126:dbl)
            n725 = case shown="False" "W/ Offset 2" {
              tunnel: w1127 -> [_ w1134]
              tunnel: w1126 -> [_ w1133]
              tunnel: w1125 -> [w1129 _]
              frame False {
                n726 = case shown="False" w1129 {
                  frame False {
                    n727 = Multiply(x="Cal read wait (s)", y=u32 1000 ("milliseconds to wait")) -> (x*y=w1131:u32)
                    n728 = Wait (ms)(milliseconds to wait=w1131) -> ()  [unwired: 1 out]
                  }
                  frame True {
                  }
                }
              }
              frame True {
                n729 = stacked-sequence {
                  tunnel: w1134 -> [_ _ _ _ _ _ _ _ _ w1155 _ _]
                  tunnel: w1133 -> [_ _ _ _ _ _ _ _ _ w1153 _ _]
                  frame #0 {
                    n730 = property on="Save ave N" class="DigNum (strict)"("Val(Sgnl)"=1.0 ("Value (Signaling)")) -> ()  [unwired: 2 in, 2 out]
                  }
                  frame #1 {
                    n731 = Wait (ms)(milliseconds to wait=u32 500) -> ()  [unwired: 1 out]
                  }
                  frame #2 {
                    n732 = property on="Trap Delta (MHz)" class="DigNum (strict)"("Val(Sgnl)"="Offset 2 Start (MHz)") -> ()  [unwired: 2 in, 2 out]
                    n733 = Replace Array Subset(array=u32[] [0] ("Index Values"), new element="Offset 2 Set", index=0) -> (w1139:u32[])
                    n734 = property on="Saved AOD Raster Scan Parameter Sets" class="Arr (strict)"("Index Values"=w1139) -> ()  [unwired: 2 in, 2 out]
                  }
                  frame #3 {
                    n735 = Wait (ms)(milliseconds to wait=u32 500) -> ()  [unwired: 1 out]
                  }
                  frame #4 {
                    n736 = property on="Load parameters" class="Bool (strict)"("Val(Sgnl)"=TRUE ("Value (Signaling)")) -> ()  [unwired: 2 in, 2 out]
                  }
                  frame #5 {
                    n737 = Wait (ms)(milliseconds to wait=u32 500) -> ()  [unwired: 1 out]
                  }
                  frame #6 {
                    n738 = property on="Trap Raster Scan" class="Bool (strict)"("Val(Sgnl)"=TRUE ("Value (Signaling)")) -> ()  [unwired: 2 in, 2 out]
                  }
                  frame #7 {
                    n739 = Wait (ms)(milliseconds to wait=u32 2000) -> ()  [unwired: 1 out]
                  }
                  frame #8 {
                    n740 = while {
                      stop <- w1148 stop-if-true
                      n741 = local read "Raster Scanning..."() -> (w1151:bool)
                      n742 = local read "Saving..."() -> (w1149:bool)
                      n743 = Wait (ms)(milliseconds to wait=u32 100) -> ()  [unwired: 1 out]
                      n744 = Not(x=w1149) -> (.not. x?=w1147:bool)
                      n745 = Not(x=w1151) -> (.not. x?=w1150:bool)
                      n746 = And(x=w1150, y=w1147) -> (x .and. y?=w1148:bool)
                    }
                  }
                  frame #9 {
                    n747 = property on="Trap Delta (MHz)" class="DigNum (strict)"("Val(Sgnl)"=w1155) -> ()  [unwired: 2 in, 2 out]
                    n748 = property on="Saved AOD Raster Scan Parameter Sets" class="Arr (strict)"("Index Values"=u32[] [0]) -> ()  [unwired: 2 in, 2 out]
                    n749 = property on="Save ave N" class="DigNum (strict)"("Val(Sgnl)"=w1153) -> ()  [unwired: 2 in, 2 out]
                  }
                  frame #10 {
                    n750 = Wait (ms)(milliseconds to wait=u32 500) -> ()  [unwired: 1 out]
                  }
                  frame #11 {
                    n751 = property on="Load parameters" class="Bool (strict)"("Val(Sgnl)"=TRUE ("Value (Signaling)")) -> ()  [unwired: 2 in, 2 out]
                  }
                }
              }
            }
          }
          frame #9 {
            n752 = property on="Read Cal" class="Bool (strict)"("Val(Sgnl)"=TRUE ("Value (Signaling)")) -> ()  [unwired: 2 in, 2 out]
          }
          frame #10 {
            n753 = Wait (ms)(milliseconds to wait=u32 1000) -> ()  [unwired: 1 out]
          }
          frame #11 {
            n754 = property on="Fish for Tether" class="Bool (strict)"("Val(Sgnl)"=TRUE ("Value (Signaling)")) -> ()  [unwired: 2 in, 2 out]
          }
        }
        n755 = local write "Cal/Data Acq. Spot"(FALSE ("Cal/Data Acq. Spot")) -> ()
      }
      event "Dump Beads": Value Change {
        n756 = event-data() -> ()  [unwired: 1 in, 5 out]
        n757 = flat-sequence {
          tunnel: ["Dump spot flow on?"] -> w1161
          tunnel: [w1172] -> w1162
          tunnel: w1161 -> [w1172]
          tunnel: w1165 -> [w1177]
          tunnel: w1164 -> [w1176]
          tunnel: [w1174] -> w1163
          tunnel: w1162 -> [w1174]
          tunnel: w1163 -> [w1187]
          frame #0 {
            w1166 = FALSE ("Value (Signaling)")
            n758 = local read "Saving..."() -> (w1168:bool)
            n759 = local write "Dump Beads"(FALSE ("Dump Beads")) -> ()
            n760 = property on="Inject Pump 3" class="Bool (strict)"("Val(Sgnl)"=w1166) -> ()  [unwired: 2 in, 2 out]
            n761 = property on="Inject Pump 1" class="Bool (strict)"("Val(Sgnl)"=w1166) -> ()  [unwired: 2 in, 2 out]
            n762 = local write "Stop Saving"(w1168) -> ()
          }
          frame #1 {
            w1169 = FALSE ("Fl. Triggered...")
            n763 = case shown="True" "Dump spot flow on?" {
              frame False {
              }
              frame True {
                n764 = property on="Sample Channel\nFlow" class="Bool (strict)"("Val(Sgnl)"=TRUE ("Stage Moving")) -> ()  [unwired: 2 in, 2 out]
              }
            }
            n765 = local write "Fl. Triggered..."(w1169) -> ()
            n766 = local write "Tether"(w1169) -> ()
            n767 = property on="Green Laser ON/Interlacing" class="Bool (strict)"("Val(Sgnl)"=w1169) -> ()  [unwired: 2 in, 2 out]
            n768 = property on="Trap Pos. FB ON" class="Bool (strict)"("Val(Sgnl)"=w1169) -> ()  [unwired: 2 in, 2 out]
            n769 = property on="Trap Trig. Fl." class="Bool (strict)"("Val(Sgnl)"=w1169) -> ()  [unwired: 2 in, 2 out]
            n770 = property on="Fl. Triggered..." class="Bool (strict)"("Val(Sgnl)"=w1169) -> ()  [unwired: 2 in, 2 out]
            n771 = property on="Dip for Protein" class="Bool (strict)"("Val(Sgnl)"=w1169) -> ()  [unwired: 2 in, 2 out]
            n772 = property on="Pause dwell" class="Bool (strict)"("Val(Sgnl)"=w1169) -> ()  [unwired: 2 in, 2 out]
          }
          frame #2 {
            n773 = property on="Trap Pos. FB Offset Factor" class="DigNum (strict)"("Val(Sgnl)"=i64 0 ("Value (Signaling)")) -> ()  [unwired: 2 in, 2 out]
          }
          frame #3 {
            n774 = local read "Saved Stage Positions"() -> (w1178:dbl[][])
            n775 = local write "Stage Moving"(TRUE ("Stage Moving")) -> ()
            n776 = Array Subset(array=w1178, index (row)=3 ("index"), length (row)=1 ("length"), index (col)=1 ("index"), length (col)=3 ("length")) -> (w1183:dbl[][])
            n777 = Reshape Array(w1183, 3 ("dimension size")) -> (w1181:dbl[])
            n778 = Array To Cluster(array=w1181) -> (cluster=w1180:cluster{"[0]":dbl, "[1]":dbl, "[2]":dbl})
            n779 = call "Set Stage Position.vi"("Position"=w1180, "error in"=w1176, "VISA resource name in"=w1177) -> ()  [unwired: 3 out]
          }
          frame #4 {
            w1188 = FALSE ("Value (Signaling)")
            n780 = case shown="True" w1187 {
              frame False {
              }
